vi "svx_SC Line Update Pair.vi"(6 "State in":T1={"X Scale"={"Name"="Horizontal", "format string"="%#.2g", "Major Color"=16777238, "Minor Color"=16777216, "Scale Visible"=TRUE, " Label Visible"=TRUE, "Grid Style"=1, "Maximum"=1.0, "Minimum"=-1.0}, "Y Scale"={"Name"="Vertical", "format string"="%#.2g", "Major Color"=16777238, "Minor Color"=16777216, "Scale Visible"=TRUE, " Label Visible"=TRUE, "Grid Style"=1, "Maximum"=1.0, "Minimum"=-1.0}, "Plot"={"Point Style"=0, "Line Width"=0, "Line Style"=0, "Plot Color"=16860, "Point/fill"=16860}, "Arrow Color"=16860, "Autoscale"=TRUE, "Property Name"=[], "Container Bounds"={"Width"=550, "Height"=313}, "Background color"=16777226, "Annotation List"=[], "Cursor"={"Cursor Point Style"=13, "Cursor Style"=4, "Cursor Line Width"=1, "Cursor Line Style"=0, "Cursor Color"=16711680, "Cursor Name Visible"=TRUE, "Cursor Visible"=TRUE, "Cursor Position"={"X"=0.0, "Y"=0.0}, "Cursor Index"=0, "Lock Cursor Name"=FALSE, "Cursor reference"=0.0}, "size"=0, "Boundary Color"=9868950, "Maximum"=1.0, "Marker Point Style"=2, "Maker Visible"=TRUE, "Marker Color"=16860, "pair strings []"=[], "clearance boundary"=[{"boundary"={"x axis"=0.0, "y axis"=0.0}, "start point"=enum."center"}], "Custom pair name"=FALSE, "selector.visible"=TRUE, "Cursor Release"=refnum, "Children Tags"=[], "open?"=TRUE, "pair index"=[], "Legend Width"=200, " Parents Tags"="", "Label"="", "Legend Background"=16777226, "Legend Font"=16777222, "scale fit"=2, "user strings []"=[], "Item Width"=0, "out of state queue"=refnum, "property nodes"=refnum, "Kind"=enum."X-Scale", "Scale Range Change"=refnum} caption="State" {"pair index" min=0}, 10 "Label.Text":string, 11 "shaft centerline":T5) -> (0 "update tree?":bool, 4 "State out":T1={"X Scale"={"Name"="Horizontal", "format string"="%#.2g", "Major Color"=16777238, "Minor Color"=16777216, "Scale Visible"=TRUE, " Label Visible"=TRUE, "Grid Style"=1, "Maximum"=1.0, "Minimum"=-1.0}, "Y Scale"={"Name"="Vertical", "format string"="%#.2g", "Major Color"=16777238, "Minor Color"=16777216, "Scale Visible"=TRUE, " Label Visible"=TRUE, "Grid Style"=1, "Maximum"=1.0, "Minimum"=-1.0}, "Plot"={"Point Style"=0, "Line Width"=0, "Line Style"=0, "Plot Color"=16860, "Point/fill"=16860}, "Arrow Color"=16860, "Autoscale"=TRUE, "Property Name"=[], "Container Bounds"={"Width"=550, "Height"=313}, "Background color"=16777226, "Annotation List"=[], "Cursor"={"Cursor Point Style"=13, "Cursor Style"=4, "Cursor Line Width"=1, "Cursor Line Style"=0, "Cursor Color"=16711680, "Cursor Name Visible"=TRUE, "Cursor Visible"=TRUE, "Cursor Position"={"X"=0.0, "Y"=0.0}, "Cursor Index"=0, "Lock Cursor Name"=FALSE, "Cursor reference"=0.0}, "size"=0, "Boundary Color"=9868950, "Maximum"=1.0, "Marker Point Style"=2, "Maker Visible"=TRUE, "Marker Color"=16860, "pair strings []"=[], "clearance boundary"=[{"boundary"={"x axis"=0.0, "y axis"=0.0}, "start point"=enum."center"}], "Custom pair name"=FALSE, "selector.visible"=TRUE, "Cursor Release"=refnum, "Children Tags"=[], "open?"=TRUE, "pair index"=[], "Legend Width"=200, " Parents Tags"="", "Label"="", "Legend Background"=16777226, "Legend Font"=16777222, "scale fit"=2, "user strings []"=[], "Item Width"=0, "out of state queue"=refnum, "property nodes"=refnum, "Kind"=enum."X-Scale", "Scale Range Change"=refnum} caption="State" {"pair index" min=0})   [LabVIEW 2017, in "SVX SC Line.xctl"]
uses:
  <vilib>/addons/_XControls/Shaft Centerline/SVX SC Line.xctl
  <vilib>/addons/_XControls/Shaft Centerline/subVIs/svx_SC Line Data.ctl
  <vilib>/addons/_XControls/Shaft Centerline/subVIs/svx_SC Line State.ctl
  <vilib>/addons/_XControls/Shaft Centerline/subVIs/svx_SC Line Bounds.ctl
  <vilib>/addons/_XControls/Shaft Centerline/subVIs/svx_SC Line Annotation List.ctl
  <vilib>/addons/_XControls/Shaft Centerline/subVIs/svx_SC Line OutState Queue.ctl
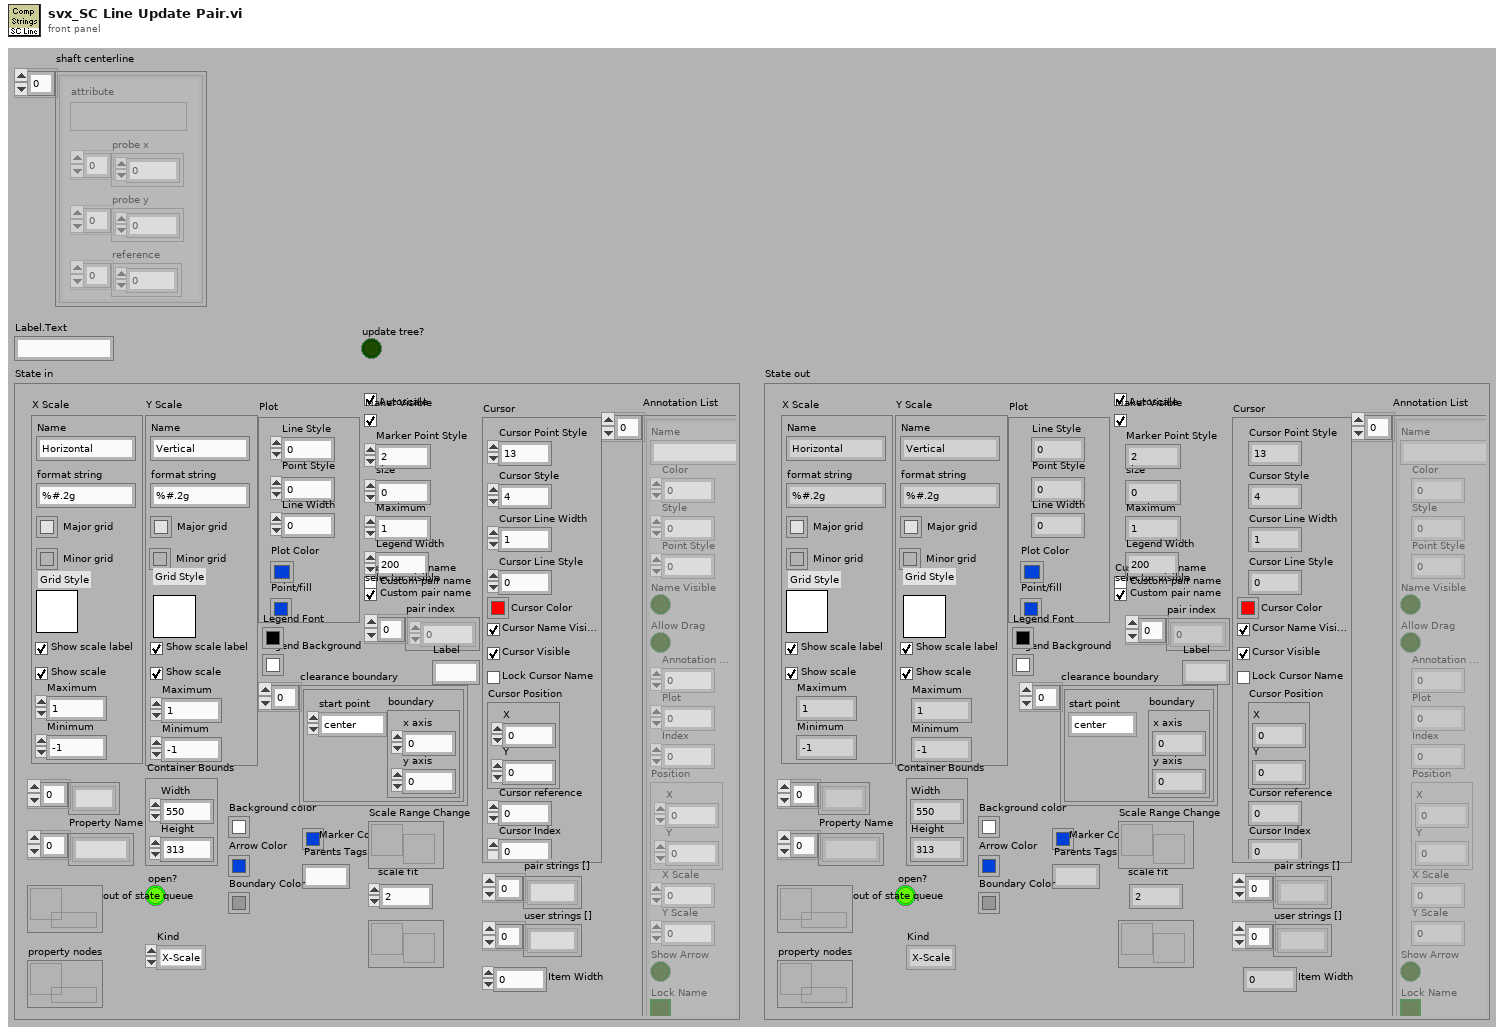
[diagram p1: front panel]
types:
  T1 = typedef "SVX SC Line.xctl/svx_SC Line State.ctl" = cluster{"X Scale":cluster{"Name":string, "format string":string, "Major Color":u32, "Minor Color":u32, "Scale Visible":bool, " Label Visible":bool, "Grid Style":u16, "Maximum":dbl, "Minimum":dbl}, "Y Scale":cluster{"Name":string, "format string":string, "Major Color":u32, "Minor Color":u32, "Scale Visible":bool, " Label Visible":bool, "Grid Style":u16, "Maximum":dbl, "Minimum":dbl}, "Plot":cluster{"Point Style":u8, "Line Width":u8, "Line Style":u8, "Plot Color":u32, "Point/fill":u32}, "Arrow Color":u32, "Autoscale":bool, "Property Name":string[], "Container Bounds":T2, "Background color":u32, "Annotation List":T3, "Cursor":cluster{"Cursor Point Style":u8, "Cursor Style":u8, "Cursor Line Width":u8, "Cursor Line Style":u8, "Cursor Color":u32, "Cursor Name Visible":bool, "Cursor Visible":bool, "Cursor Position":cluster{"X":dbl, "Y":dbl}, "Cursor Index":i32, "Lock Cursor Name":bool, "Cursor reference":dbl}, "size":i32, "Boundary Color":u32, "Maximum":dbl, "Marker Point Style":u8, "Maker Visible":bool, "Marker Color":u32, "pair strings []":string[], "clearance boundary":cluster{"boundary":cluster{"x axis":dbl, "y axis":dbl}, "start point":enum16{"center", "top", "bottom"}}[], "Custom pair name":bool, "selector.visible":bool, "Cursor Release":refnum<user-event>, "Children Tags":string[], "open?":bool, "pair index":i32[], "Legend Width":u32, " Parents Tags":string, "Label":string, "Legend Background":u32, "Legend Font":u32, "scale fit":u8, "user strings []":string[], "Item Width":u32, "out of state queue":T4, "property nodes":refnum<queue>, "Kind":enum16{"X-Scale", "Y-Scale", "Z-Scale"}, "Scale Range Change":refnum<user-event>}
  T2 = typedef "SVX SC Line.xctl/svx_SC Line Bounds.ctl" = cluster{"Width":u32, "Height":u32}
  T3 = typedef "SVX SC Line.xctl/svx_SC Line Annotation List.ctl" = cluster{"Name":string, "Color":u32, "Style":u8, "Point Style":u8, "Name Visible":bool, "Allow Drag":bool, "Annotation Mode":u32, "Plot":i32, "Index":i32, "Position":cluster{"X":dbl, "Y":dbl}, "X Scale":u32, "Y Scale":u32, "Show Arrow":bool, "Lock Name":bool, "Plot Area":i32, "Label Offset":cluster{"X":dbl, "Y":dbl}}[]
  T4 = typedef "SVX SC Line.xctl/svx_SC Line OutState Queue.ctl" = refnum<queue>
  T5 = typedef "SVX SC Line.xctl/svx_SC Line Data.ctl" = cluster{"probe x":dbl[], "probe y":dbl[], "reference":dbl[], "attribute":variant}[]
  T6 = cluster{"boundary":cluster{"x axis":dbl, "y axis":dbl}, "start point":enum16{"center", "top", "bottom"}}[]
  T7 = cluster{"boundary":cluster{"x axis":dbl, "y axis":dbl}, "start point":enum16{"center", "top", "bottom"}}
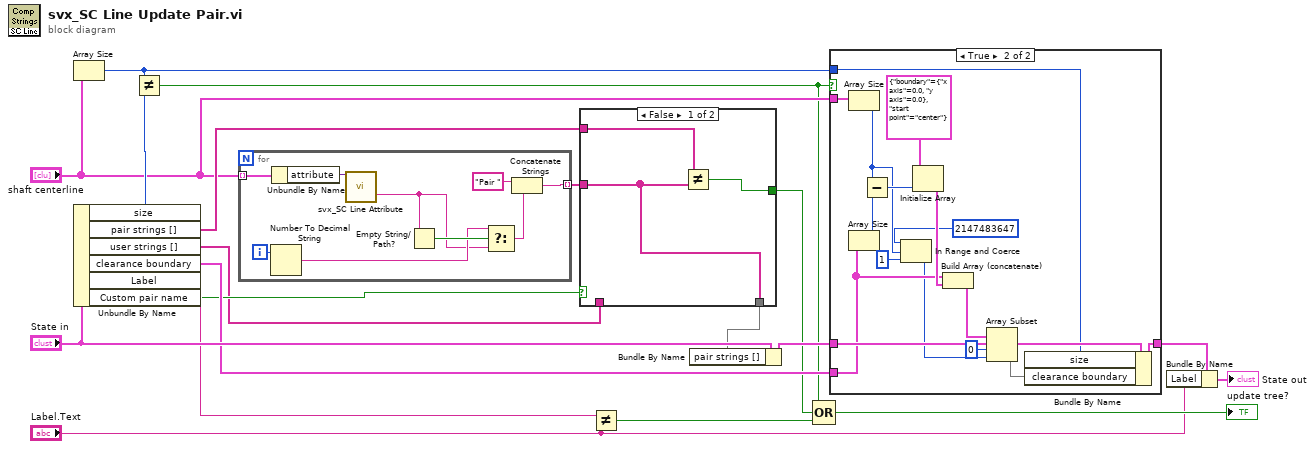
[diagram p0: block diagram]
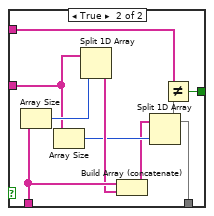
[diagram p2: hidden frame]
diagram:
  n1 = Array Size(array="shaft centerline") -> (size(s)=w13:i32)
  n2 = Unbundle By Name("State in") -> ("size"=w14:i32, "pair strings []"=w5:string[], "user strings []"=w6:string[], "clearance boundary"=w12:T6, "Label"=w17:string, "Custom pair name"=w8:bool)
  n3 = Not Equal?(x=w13, y=w14) -> (x != y?=w1:bool)
  n4 = for {
    tunnel: "shaft centerline" -> [w27] mode=indexing
    tunnel: [w24] -> w7 mode=indexing
    i -> [w28]
    n5 = Number To Decimal String(number=w28) -> (decimal integer string=w21:string)  [unwired: 1 in]
    n6 = Unbundle By Name(w27) -> ("attribute"=w23:variant)
    n7 = call <vilib>:"svx_SC Line Attribute.vi"("attribute"=w23) -> ("pair"=w20:string)  [unwired: 14 in, 4 out]
    n8 = Empty String/Path?(string/path=w20) -> (empty?=w22:bool)
    n9 = Select(t=w21, s=w22, f=w20) -> (s? t:f=w25:string)
    n10 = Concatenate Strings("Pair " ("string"), w25) -> (w24:string)
  }
  n11 = case shown="False" w8 {
    tunnel: w7 -> [w29 w39]
    tunnel: w6 -> [_ w38]
    tunnel: w5 -> [w31 w34]
    tunnel: [w30 w33] -> w4
    tunnel: [w29 w32] -> w3
    frame False {
      n12 = Not Equal?(x=w31, y=w29) -> (x != y?=w30:bool)
    }
    frame True {
      n13 = Array Size(array=w38) -> (size(s)=w40:i32)
      n14 = Array Size(array=w39) -> (size(s)=w36:i32)
      n15 = Split 1D Array(array=w39, index=w40) -> (second subarray=w37:string[])  [unwired: 1 out]
      n16 = Build Array (concatenate)(w38, w37) -> (w35:string[])
      n17 = Split 1D Array(array=w35, index=w36) -> (first subarray=w32:string[])  [unwired: 1 out]
      n18 = Not Equal?(x=w34, y=w32) -> (x != y?=w33:bool)
    }
  }
  n19 = Not Equal?(x=w17, y="Label.Text") -> (x != y?=w16:bool)
  n20 = Bundle By Name(cluster="State in", "pair strings []"=w3) -> (w18:T1)
  n21 = Compound Arithmetic op=OR(w1, w4, w16) -> (→"update tree?":bool)
  n22 = case shown="True" w1 {
    tunnel: [w41 w55] -> w11
    tunnel: w18 -> [w41 w49]
    tunnel: "shaft centerline" -> [_ w48]
    tunnel: w13 -> [_ w47]
    tunnel: w12 -> [_ w46]
    frame False {
    }
    frame True {
      n23 = Array Size(array=w48) -> (size(s)=w45:i32)
      n24 = Array Size(array=w46) -> (size(s)=w53:i32)
      n25 = Subtract(x=w45, y=w53) -> (x-y=w57:i32)
      n26 = In Range and Coerce(upper limit=2147483647 ("lower limit"), x=w45, lower limit=1) -> (coerced(x)=w43:i32)  [unwired: 1 out]
      n27 = Initialize Array(T7 {"boundary"={"x axis"=0.0, "y axis"=0.0}, "start point"=enum."center"} ("clearance boundary settings"), w57) -> (w56:T6)
      n28 = Build Array (concatenate)(w46, w56) -> (w54:T6)
      n29 = Array Subset(array=w54, index=0, length=w43) -> (w52:T6)
      n30 = Bundle By Name(cluster=w49, "size"=w47, "clearance boundary"=w52) -> (w55:T1)
    }
  }
  n31 = Bundle By Name(cluster=w11, "Label"="Label.Text") -> (→"State out":T1)
